vi "Optics_SetRelativePosition.VI"(8 "Error in":errorcluster, 9 "Position":dbl, 10 "Motor":dbl, 11 "VISA in":refnum<visa-resource-name>) -> (0 "Error out":errorcluster, 3 "VISA out":refnum<visa-resource-name>)   [LabVIEW 2021]
panel:
  out "String sent":string
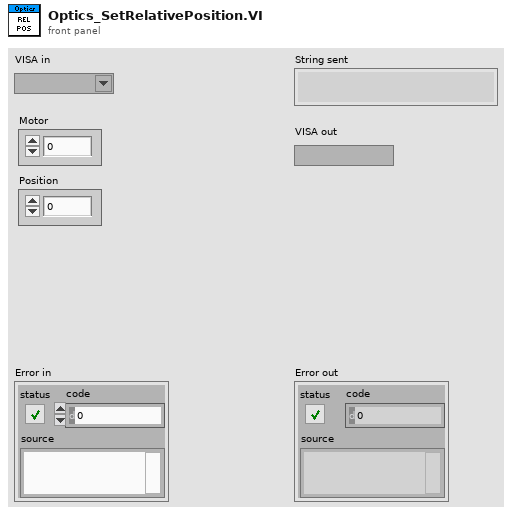
[diagram p1: front panel]
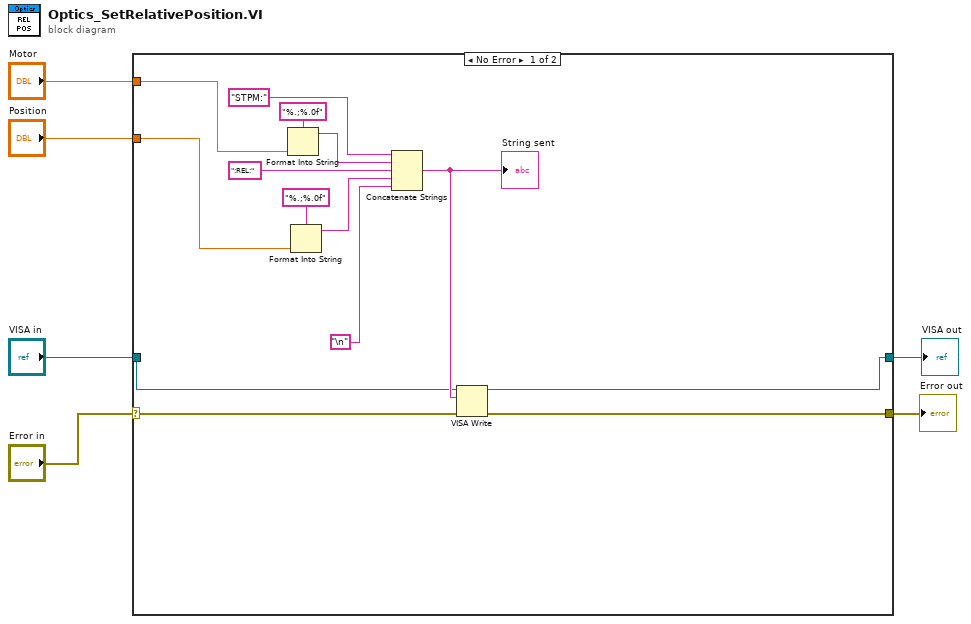
[diagram p0: block diagram]
diagram:
  n1 = case shown="No Error" "Error in" {
    selector: "Error in" -> [w10 w22]
    tunnel: [w9 w22] -> w6
    tunnel: "Motor" -> [w17 _]
    tunnel: "Position" -> [w16 _]
    tunnel: "VISA in" -> [w7 w21]
    tunnel: [w8 w21] -> w1
    frame No Error {
      n2 = Format Into String(format string="%.;%.0f", w17) -> (resulting string=w20:string)  [unwired: 2 in, 1 out]
      n3 = Format Into String(format string="%.;%.0f", w16) -> (resulting string=w15:string)  [unwired: 2 in, 1 out]
      n4 = Concatenate Strings("STPM:", w20, ":REL:", w15, "\n") -> (w11:string)
      "String sent" <- w11
      n5 = VISA Write(VISA resource name=w7, write buffer=w11, error in (no error)=w10) -> (VISA resource name out=w8:refnum<visa-resource-name>, error out=w9:errorcluster)  [unwired: 1 out]
    }
    frame Default {
    }
  }
  "Error out" <- w6
  "VISA out" <- w1
